vi "Specific Enthalpy Difference of Pure Water (J to kg).vi"(1 "Lower Temp Water":dbl[unit], 2 "Higher Temp Water":dbl[unit]) -> (0 "Specific Enthalpy Difference":dbl[unit])   [LabVIEW 2018]
panel:
  out "Lower Enthalphy of Pure Water":dbl[unit]
  out "Higher Enthalphy of Pure Water":dbl[unit]
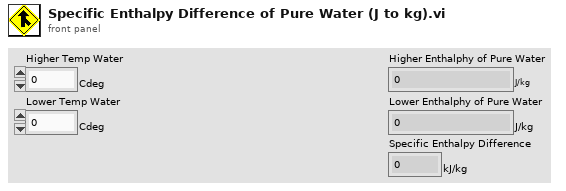
[diagram p1: front panel]
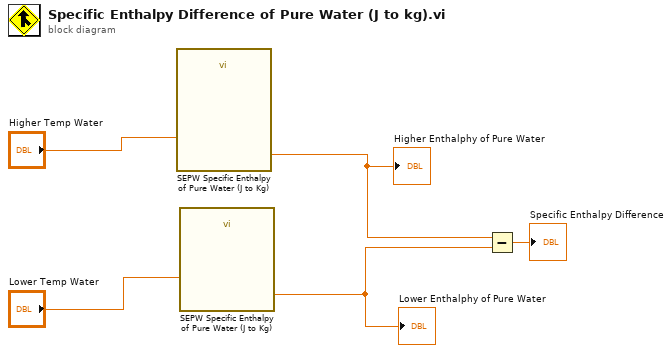
[diagram p0: block diagram]
diagram:
  n1 = call "SEPW Specific Enthalpy of Pure Water (J to Kg).vi"("Temp Pure Wate"="Higher Temp Water") -> ("SEPW"=w3:dbl[unit])
  "Higher Enthalphy of Pure Water" <- w3
  n2 = call "SEPW Specific Enthalpy of Pure Water (J to Kg).vi"("Temp Pure Wate"="Lower Temp Water") -> ("SEPW"=w2:dbl[unit])
  "Lower Enthalphy of Pure Water" <- w2
  n3 = Subtract(x=w3, y=w2) -> (x-y=→"Specific Enthalpy Difference":dbl[unit])
